vi "VA CoAP - Very basic Test.vi"() -> ()   [LabVIEW 2020]
uses:
  <vilib>/httpClient/LabVIEWHTTPClient.lvlib
panel:
  out "headers":string
  out "body":string
  out "error out":errorcluster
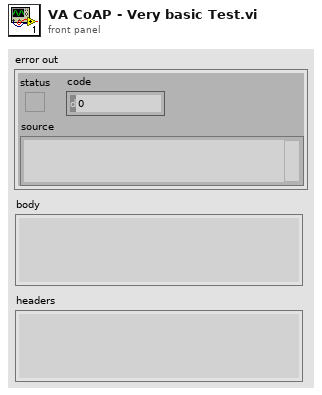
[diagram p1: front panel]
types:
  T1 = typedef "LabVIEWHTTPClient.lvlib/ClientHandle.ctl" = refnum<k1>
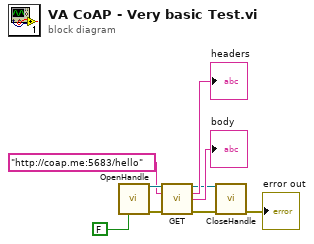
[diagram p0: block diagram]
diagram:
  n1 = call <vilib>:"OpenHandle.vi"("verify server(true)"=FALSE) -> ("client handle out"=w4:T1, "error out"=w3:errorcluster)  [unwired: 13 in]
  n2 = call <vilib>:"GET.vi"("client handle"=w4, "url"="http://coap.me:5683/hello", "error in (no error)"=w3) -> ("client handle out"=w1:T1, "headers"=→"headers":string, "body"=→"body":string, "error out"=w9:errorcluster)  [unwired: 9 in]
  n3 = call <vilib>:"CloseHandle.vi"("client handle"=w1, "error in (no error)"=w9) -> ("error out"=→"error out":errorcluster)  [unwired: 13 in]
